vi "fgv_look-ahead_config.vi"(7 "cmd":enum16{"read", "write"}(ring), 11 "lookahed cfg in":T2={"lookahead pt n"=64.0, "lookahead distance "=2.0}) -> (3 "lookahed cfg out":T1={"lookahead pt n"=64.0, "lookahead distance"=2.0})   [LabVIEW 2019]
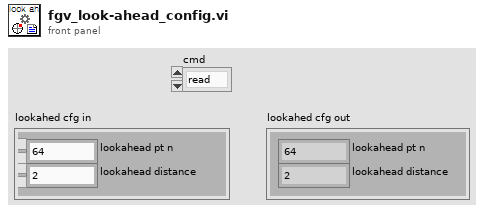
[diagram p1: front panel]
types:
  T1 = cluster{"lookahead pt n":dbl, "lookahead distance":dbl}
  T2 = cluster{"lookahead pt n":dbl, "lookahead distance ":dbl}
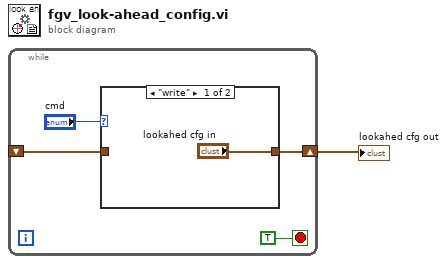
[diagram p0: block diagram]
diagram:
  n1 = while {
    shift-right: [w4] -> w1
    shift-left: _ -> [w3]
    stop <- TRUE stop-if-true
    n2 = case shown="\"write\"" "cmd" {
      tunnel: ["lookahed cfg in" w7] -> w4
      tunnel: w3 -> [_ w7]
      frame "write" {
      }
      frame "read", Default {
      }
    }
  }
  "lookahed cfg out" <- w1
